vi "FilterTwoCurves.vi"(0 "high cut-off freq":i32=19, 2 "ForceSignal":dbl[](array[numeric]), 3 "filter on-off":enum32{"filter", "no filter"}(ring), 4 "low cut-off freq":i32=25, 5 "order":i32=4 step=1, 6 "Fsampling":i32=2000, 7 "filter type":T1(ring)) -> (1 "Filtered":dbl[](graph))   [LabVIEW 2010]
uses:
  <vilib>/Analysis/3filter.llb/Butterworth Filter (DBL).vi
  <vilib>/Analysis/NI_AALBase.lvlib
panel:
  out "Raw":dbl[](graph)
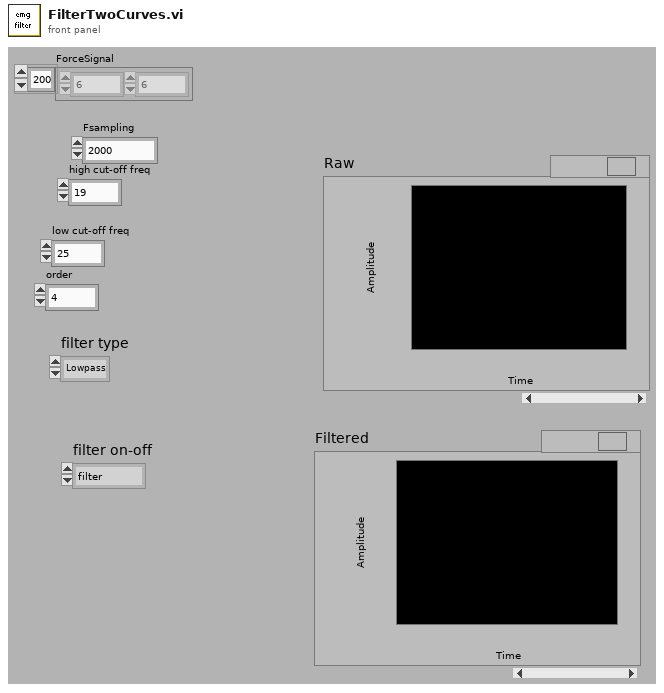
[diagram p1: front panel]
types:
  T1 = enum32{"Lowpass", "Highpass", "Bandpass", "Bandstop"}
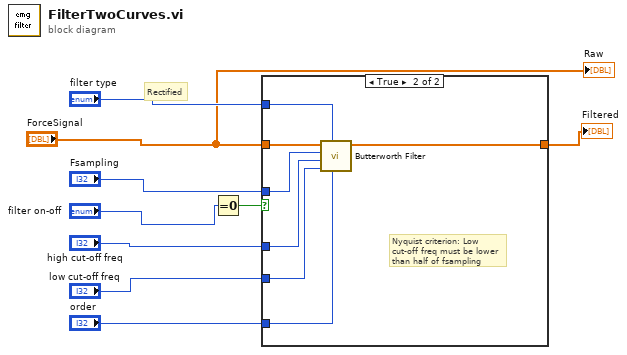
[diagram p0: block diagram]
diagram:
  # "Rectified"
  n1 = Equal To 0?(x="filter on-off") -> (x = 0?=w2:bool)
  n2 = case shown="True" w2 {
    tunnel: "Fsampling" -> [_ w17]
    tunnel: "filter type" -> [_ w16]
    tunnel: "high cut-off freq" -> [_ w15]
    tunnel: "low cut-off freq" -> [_ w14]
    tunnel: "order" -> [_ w13]
    tunnel: [w10 w11] -> w3
    tunnel: "ForceSignal" -> [w10 w12]
    frame False {
    }
    frame True {
      # "Nyquist criterion: Low \ncut-off freq must be lower than half of fsampling"
      n3 = call-poly <vilib>:"Butterworth Filter.vi"("order"=w13, "filter type"=w16, "low cutoff freq: fl"=w14, "high cutoff freq: fh"=w15, "sampling freq: fs"=w17, "X"=w12) -> ("Filtered X"=w11:dbl[])  [unwired: 2 in, 1 out]
    }
  }
  "Filtered" <- w3
  "Raw" <- "ForceSignal"
